vi "SVT Phase Linearity (1 Ch).vi"(0 "scaled signal [EU]":waveform(dbl)={"t0"=timestamp(0 s since 1904-01-01), "dt"=0.0, "Y"=[]}, 2 "frequency range":T9={"start frequency"=-1.0, "stop frequency"=-1.0} {"stop frequency" format="%.2f"; "start frequency" format="%.2f"}, 3 "magnitude threshold [dB]":dbl format="%.2f", 5 "error in (no error)":errorcluster, 6 "desired units":T8) -> (11 "phase deviation spectrum":cluster{"frequencies":dbl[], "phases":dbl[]}(graph), 12 "unit labels":T7, 13 "average group delay":dbl=nan format="%.2f", 14 "magnitude spectrum":cluster{"f0":dbl, "df":dbl, "magnitude":dbl[]}(graph), 15 "phase spectrum":cluster{dbl[], dbl[]}[](graph), 16 "max phase deviation":dbl=nan format="%.3p", 17 "multitone phase":cluster{"frequency [Hz]":dbl, "phase":dbl}[](array[cluster]) {"phase" format="%.2f"; "frequency [Hz]" format="%.2f"}, 18 "spectrum info":T1={"channel name"="", "description"="", "x-axis units"=0, "spectral info"={"spectrum type"=enum."Power [Magnitude^2]", "linear/dB"=enum."linear", "window"=0, "window size"=0, "FFT size"=0}, "engineering units"=0, "custom label"="", "dB reference [EU]"=0.0, "peak units"=enum."rms", "weighting filter"=0, "spectral density?"=FALSE, "unit label"="", "spectrum skewed?"=FALSE, "complimentary spectrum units"=enum."none"} {"x-axis units" items=["Time (s)"=0, "Frequency-CB (Hz)"=1, "Frequency-CPB (Hz)"=1248, "Frequency-Arbitrary (Hz)"=2357, "Quefrency (s)"=2, "Revolutions (rev)"=3, "Order"=4, "Speed (RPM)"=11, "Speed (rad/s)"=21, "Index"=65535]; "weighting filter" items=["Linear", "A-weighting", "B-weighting", "C-weighting", "ITU-R 468-4", "Dolby", "CCITT", "C-message", "Wb", "Wc", "Wd", "We", "Wf", "Wh", "Wj", "Wk", "Wm", "AES17 20 kHz lowpass", "AES17 40 kHz lowpass", "AES17 20 kHz highpass", "AES17 40 kHz highpass"]; "dB reference [EU]" format="%.2f"; "engineering units" items=["custom..."=0, "V"=1, "A"=21, "C"=30, "pC"=31, "s"=32, "-"=29, "Pa"=2, "N"=20, "g"=3, "m/s^2"=4, "m/s"=5, "m"=6, "mm/s"=12, "mm"=13, "micron/s"=14, "micron"=15, "in/s^2"=7, "in/s"=8, "in"=9, "mil/s"=10, "mil"=11, "rad/s^2"=16, "rad/s"=17, "rad"=18, "deg/s^2"=26, "deg/s"=27, "deg"=28, "RPM"=22, "cycle/s^2"=23, "Hz"=24, "cycle"=25, "strain"=19]; "spectral info"."window" items=["None "=0, "Hanning"=1, "Hamming"=2, "Blackman-Harris"=3, "Exact Blackman"=4, "Blackman"=5, "Flat Top"=6, "4 Term B-Harris "=7, "7 Term B-Harris"=8, "Low Sidelobe"=9, "Force - Exponential"=10, "Gaussian"=62]}, 19 "error out":errorcluster)   [LabVIEW 2017, in "SoundVib_Distortion.lvlib"]
doc: "Computes the <B>multitone phase</B> of each tone in a multitone signal, the <B>average group delay</B>, and the <B>max deviation of the phase</B> from a straight line. Use a square wave or construct the input signal with component tones evenly spaced in frequency and with zero relative phase between the component tones."
uses:
  <vilib>/addons/Sound and Vibration/svt_Distortion/SoundVib_Distortion.lvlib
  <vilib>/addons/_NISVFA/_Shared subVIs/Controls/svc_Spectrum Info.ctl
  <vilib>/addons/_NISVFA/_Shared subVIs/Controls/svc_X-Axis Units.ctl
  <vilib>/addons/_NISVFA/_Shared subVIs/Controls/svc_Spectrum Type.ctl
  <vilib>/addons/_NISVFA/_Shared subVIs/Controls/svc_Engineering Units Text Ring.ctl
  <vilib>/addons/_NISVFA/_Shared subVIs/Controls/svc_Weighting Filter Text Ring.ctl
  <vilib>/addons/_NISVFA/_Shared subVIs/Controls/svc_Complimentary Spectrum Units.ctl
  <vilib>/addons/_NISVFA/_Spectrum Processing/SVFA Get Spectrum Subset (1 Ch).vi
  <vilib>/addons/_NISVFA/_Spectrum Processing/SVFA Spectrum Peak Search (1 Ch).vi
  <vilib>/addons/_NISVFA/_Shared subVIs/Common/svc_Spectrum Units.vi
  <vilib>/addons/_NISVFA/_Spectrum Processing/subVIs/svfa_Spectrum Peak Search.vi
  <vilib>/addons/_NISVFA/_Spectrum Processing/subVIs/svfa_Peak Rough Search Indices.vi
  <vilib>/addons/_NISVFA/_Shared subVIs/Common/svc_Get Weighting Enum and Labels.vi
  <vilib>/addons/_NISVFA/_Shared subVIs/Common/svc_Unit Label Lexical Class.vi
  <vilib>/addons/_NISVFA/_Shared subVIs/Common/svc_Engineering Units to Unit Label.vi
  <vilib>/addons/_NISVFA/_Shared subVIs/Common/svc_Format Value (DBL).vi
  <vilib>/addons/_NISVFA/_Spectrum Processing/subVIs/svfa_Three Finger Peak Search.vi
  <vilib>/addons/_NISVFA/_Shared subVIs/Common/svc_Build Unit Label for Frequency Range.vi
  <vilib>/addons/_NISVFA/_Shared subVIs/Common/svc_Convert Frequency to Frequency String.vi
  <vilib>/addons/_NISVFA/_Shared subVIs/Common/svc_Check Frequency Range in Spectrum.vi
  <vilib>/addons/_NISVFA/_Baseband FFT/SVFA FFT Spectrum (Mag-Phase) (1 Ch).vi
panel:
  in  "magnitude or phase tab":enum32{"magnitude", "phase", "phase deviation"}(tab)
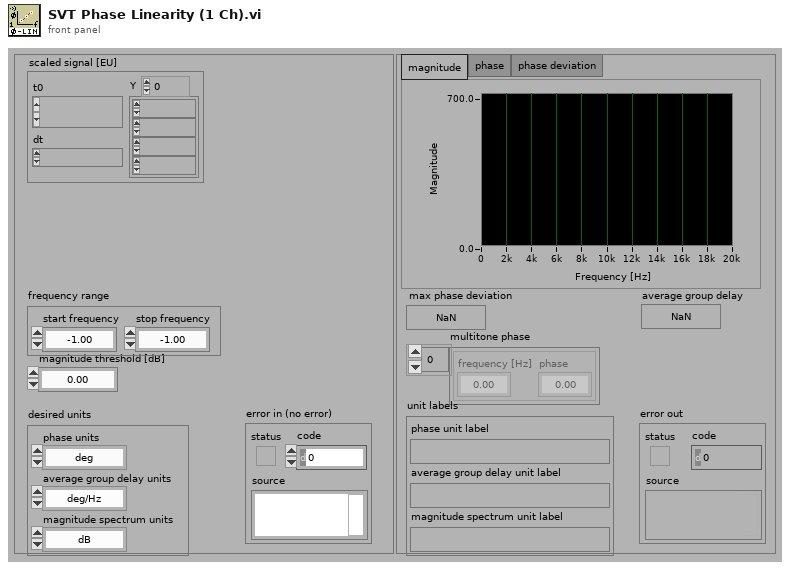
[diagram p1: front panel]
types:
  T1 = typedef "svc_Spectrum Info.ctl" = cluster{"channel name":string, "description":string, "x-axis units":T2, "spectral info":cluster{"spectrum type":T3, "linear/dB":enum16{"linear", "dB"}, "window":u16, "window size":i32, "FFT size":i32}, "engineering units":T4, "custom label":string, "dB reference [EU]":dbl, "peak units":enum16{"rms", "peak", "peak-peak"}, "weighting filter":T5, "spectral density?":bool, "unit label":string, "spectrum skewed?":bool, "complimentary spectrum units":T6}
  T2 = typedef "svc_X-Axis Units.ctl" = u16
  T3 = typedef "svc_Spectrum Type.ctl" = enum16{"FFT Spectrum [complex]", "Amplitude [Magnitude]", "Power [Magnitude^2]", "Cross Spectrum [complex]", "Frequency Response [Complex]"}
  T4 = typedef "svc_Engineering Units Text Ring.ctl" = u16
  T5 = typedef "svc_Weighting Filter Text Ring.ctl" = u16
  T6 = typedef "svc_Complimentary Spectrum Units.ctl" = enum16{"none", "radians", "degrees", "cycles", "imaginary"}
  T7 = cluster{"phase unit label":string, "average group delay unit label":string, "magnitude spectrum unit label":string}
  T8 = cluster{"phase units":enum16{"deg", "rad"}, "average group delay units":enum16{"deg/Hz", "s"}, "magnitude spectrum units":enum16{"dB", "linear"}}
  T9 = cluster{"start frequency":dbl, "stop frequency":dbl}
  T10 = cluster{"dB On (F)":bool, "unwrap phase (F)":bool, "convert to degree (T)":bool}
  T11 = cluster{"single/multiple":enum16{"Multiple Peaks", "Single Max Peak"}, "threshold":dbl}
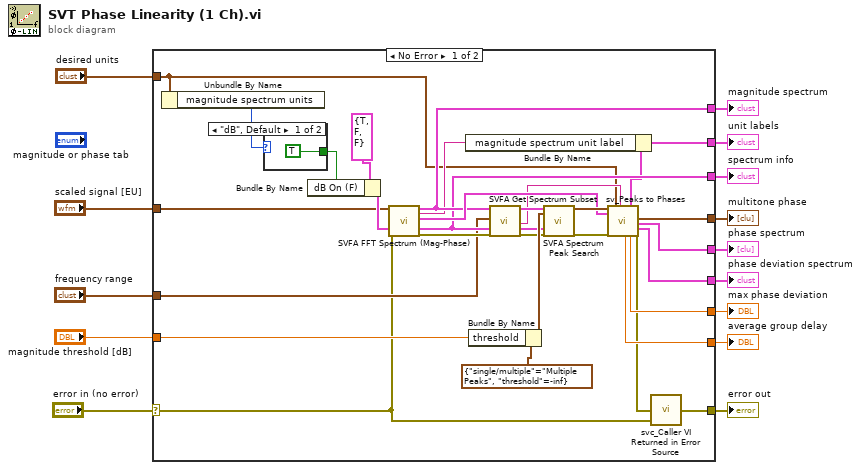
[diagram p0: block diagram]
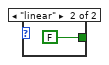
[diagram p2: hidden frame]
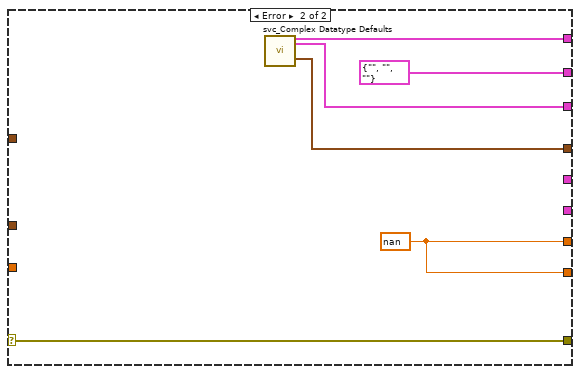
[diagram p3: hidden frame]
diagram:
  n1 = case shown="No Error" "error in (no error)" {
    selector: "error in (no error)" -> [w17 w53]
    tunnel: [w31 _] -> w14
    tunnel: [w34 w51] -> w13
    tunnel: [w20 w53] -> w12
    tunnel: "scaled signal [EU]" -> [w22 _]
    tunnel: "frequency range" -> [w19 _]
    tunnel: "magnitude threshold [dB]" -> [w40 _]
    tunnel: [w32 w50] -> w6
    tunnel: [w33 w51] -> w8
    tunnel: [w36 w49] -> w4
    tunnel: [w35 w48] -> w5
    tunnel: "desired units" -> [w15 _]
    tunnel: [w24 T7 {"phase unit label"="", "average group delay unit label"="", "magnitude spectrum unit label"=""} ("unit labels")] -> w2
    tunnel: [w16 _] -> w1
    frame No Error {
      n2 = Unbundle By Name(w15) -> ("magnitude spectrum units"=w28:enum16{"dB", "linear"})
      n3 = case shown="\"dB\", Default" w28 {
        tunnel: [TRUE ("dB On (F)") FALSE ("dB On (F)")] -> w27
        frame "dB", Default {
        }
        frame "linear" {
        }
      }
      n4 = Bundle By Name(cluster=T10 {"dB On (F)"=TRUE, "unwrap phase (F)"=FALSE, "convert to degree (T)"=FALSE} ("view"), "dB On (F)"=w27) -> (w23:T10)
      n5 = call-poly <vilib>:"SVFA FFT Spectrum (Mag-Phase).vi"("scaled signal [EU]"=w22, "view"=w23, "error in (no error)"=w17) -> ("magnitude [dB EU]"=w36:cluster{"f0":dbl, "df":dbl, "magnitude":dbl[]}, "magnitude unit label"=w26:string, "phase [degrees]"=w39:cluster{"f0":dbl, "df":dbl, "phase":dbl[]}, "spectrum info"=w35:T1, "error out"=w41:errorcluster)  [unwired: 9 in, 3 out]
      n6 = Bundle By Name(cluster=T11 {"single/multiple"=enum."Multiple Peaks", "threshold"=-inf} ("peak search settings"), "threshold"=w40) -> (w42:T11)
      n7 = call-poly <vilib>:"SVFA Get Spectrum Subset.vi"("spectrum"=w36, "range"=w19, "spectrum info"=w35, "error in (no error)"=w41) -> ("spectrum subset"=w43:cluster{"x0":dbl, "dx":dbl, "magnitude":dbl[]}, "range label"=w18:string, "dup spectrum info"=w37:T1, "error out"=w38:errorcluster)  [unwired: 10 in, 2 out]
      n8 = call-poly <vilib>:"SVFA Spectrum Peak Search.vi"("spectrum"=w43, "peak search settings"=w42, "spectrum info in"=w37, "error in (no error)"=w38) -> ("peaks"=w44:cluster{"freq. or order":dbl, "value":dbl}[], "error out"=w30:errorcluster)  [unwired: 11 in, 3 out]
      n9 = call <vilib>:"sv_Peaks to Phases.vi"("peaks"=w44, "phase [radians]"=w39, "error in"=w30, "desired units"=w15, "frequency range string"=w18) -> ("average group delay"=w33:dbl, "unit labels"=w25:T7, "maximum phase deviation"=w34:dbl, "multitone phases"=w32:cluster{"frequency":dbl, "phase":dbl}[], "phases"=w31:cluster{"frequencies":dbl[], "phases":dbl[]}[], "phase deviation"=w16:cluster{"frequencies":dbl[], "phases":dbl[]}, "error out"=w21:errorcluster)  [unwired: 6 in, 2 out]
      n10 = Bundle By Name(cluster=w25, "magnitude spectrum unit label"=w26) -> (w24:T7)
      n11 = call <vilib>:"svc_Caller VI Returned in Error Source.vi"("warning input to caller"=w17, "error in (no error)"=w21) -> ("error out"=w20:errorcluster)  [unwired: 3 in]
    }
    frame Error {
      w51 = nan
      n12 = call <vilib>:"svc_Complex Datatype Defaults.vi"() -> ("empty spectrum"=w49:cluster{"f0":dbl, "df":dbl, "magnitude":dbl[]}, "dead spectrum info"=w48:T1, "empty array of peaks"=w50:cluster{"frequency":dbl, "value":dbl}[])  [unwired: 11 in, 6 out]
    }
  }
  "phase spectrum" <- w14
  "max phase deviation" <- w13
  "error out" <- w12
  "average group delay" <- w8
  "multitone phase" <- w6
  "magnitude spectrum" <- w4
  "spectrum info" <- w5
  "unit labels" <- w2
  "phase deviation spectrum" <- w1
